vi "Get Line Count.vi"(8 "error in (no error)":errorcluster, 11 "TermBuffer in":refnum<class "TermBuffer.lvclass">) -> (0 "error out":errorcluster, 2 "Line Count":i32, 3 "TermBuffer out":refnum<class "TermBuffer.lvclass">)   [LabVIEW 2020, in "Terminal.lvlib" / "TermBuffer.lvclass"]
doc: "On scrollback buffers this will be the number of lines present in the buffer. In normal screen buffer mode this will return the current configured height of the buffer in number of rows."
uses:
  TermBuffer.lvclass
  TermBuffer.lvclass/TermBuffer.ctl
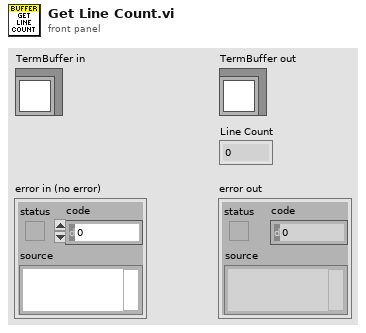
[diagram p1: front panel]
types:
  T1 = typedef "Terminal.lvlib/TermBuffer.lvclass/Ref Data.ctl" = cluster{"Lines":refnum<class "TermLine.lvclass">[], "Rows":i32, "Cols":i32}
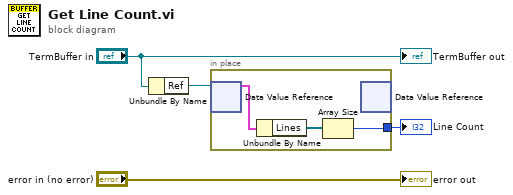
[diagram p0: block diagram]
diagram:
  n1 = Unbundle By Name("TermBuffer in") -> ("Ref"=w3:refnum<data-value>)
  n2 = in-place {
    in-place-border: [w5] -> w1
    n3 = in-place-dvr #1(w3) -> (w7:T1)  [unwired: 1 out]
    n4 = Unbundle By Name(w7) -> ("Lines"=w6:refnum<class "TermLine.lvclass">[])
    n5 = Array Size(array=w6) -> (size(s)=w5:i32)
    n6 = in-place-dvr #1() -> ()  [unwired: 1 in, 2 out]
  }
  "Line Count" <- w1
  "error out" <- "error in (no error)"
  "TermBuffer out" <- "TermBuffer in"
